vi "jrg_writeeodfile.vi"(0 "Time":string="12:00:00", 1 "Date":string="06/09/14", 2 "Path":path, 3 "Specimen":string="1", 4 "Location":string="EFish Lab", 5 "Species":string="Bennetti", 6 "UserData":sgl format="%#_13g", 7 "WaveformData":i16[](array[numeric]), 8 "NBits":i8=16, 9 "AD Range":sgl=65535.0 format="%#_13g", 10 "Version":i8, 11 "Gain":i32, 12 "NBytes":i8=2, 14 "Comments":string="Default values", 15 "Temp":string="25", 17 "Coupling":bool, 18 "Sample Rate":i32=1000, 19 "Polarity":i8) -> (13 "Path Out":path)   [LabVIEW 2014]
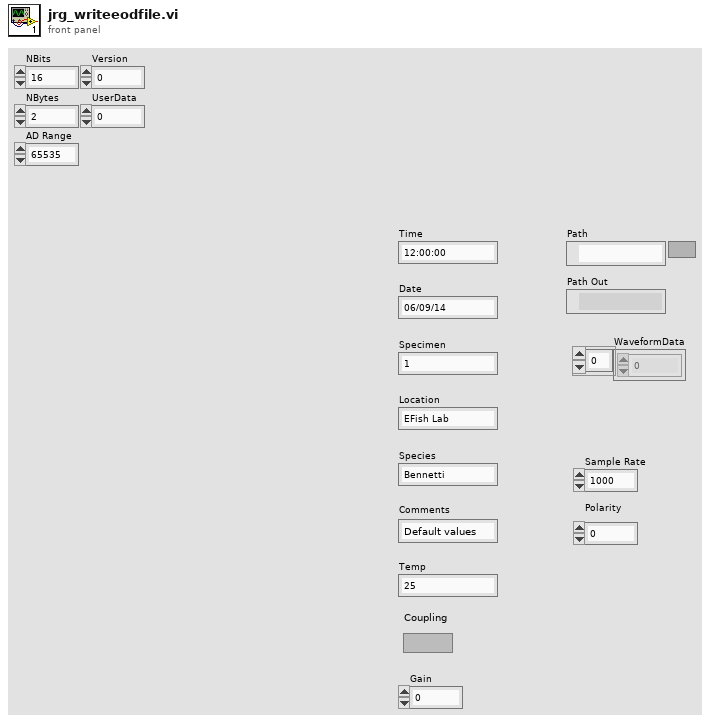
[diagram p1: front panel]
types:
  T1 = enum16{"big-endian, network order", "native, host order", "little-endian"}
  T2 = enum16{"open", "replace", "create", "open or create", "replace or create", "replace or create with confirmation"}
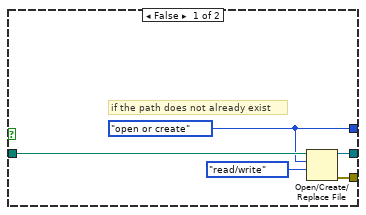
[diagram p2: hidden frame]
diagram:
  # "If File Exists,\nJump to end of file"
  # "1) If the Path is Empty:\n\na. Open file dialog\nb. Pick File Location\n\n2) If Path already exists\n\na. Open File\n\n3) If Path doesn't exist\n\na. Create File\n\n4) If Path is Full and Exists:\na. Open the file\n\n5) If Path is Full and doesn't exist\na. Create the file"
  # "Waveform Description Parameters are concatenated with prefixes:\nTime : Time of Recording\nDate: Date of Recording\nSpecimen: Specimen Number\nSpecies: Putative Species ID\nLocation: Locality Code\nComments: Further Description\nTemp: Temperature at Recording Time\nGain: Gain of Amplifier\nCoupling: AC or DC coupling\nPolarity: Inverted or Normal\n\nRecording Parameters are Gathered from Software:\nSampling Rate: Sampling Rate of A/D Converter\nNbits:\nNbytes:\nADRange:"
  n1 = Empty String/Path?(string/path="Path") -> (empty?=w22:bool)
  n2 = case shown="True" w22 {
    tunnel: "Path" -> [w34 w39]
    tunnel: [w33 w42] -> w25
    tunnel: [w32 w41] -> w27
    tunnel: [w31 w44] -> w26
    frame False {
      w31 = T2."open or create" ("operation (0:open)")
      # "if the path does not already exist"
      n3 = Open/Create/Replace File(file path (use dialog)=w34, operation (0:open)=w31, access (0:read/write)=enum16{"read/write", "read-only", "write-only"}."read/write") -> (refnum out=w33:refnum<file>, error out=w32:errorcluster)  [unwired: 3 in, 1 out]
    }
    frame True {
      # "if the path already exists"
      n4 = File Dialog(7:"Select Path", 9:"New EOD", 11:w39) -> (0:w40:errorcluster, 2:w47:bool, 3:w43:path)  [unwired: 4 in, 1 out]
      n5 = Select(t=T2."open" ("operation (0:open)"), s=w47, f=T2."create" ("operation (0:open)")) -> (s? t:f=w44:T2)
      n6 = Open/Create/Replace File(file path (use dialog)=w43, error in=w40, operation (0:open)=T2."create", access (0:read/write)=enum16{"read/write", "read-only", "write-only"}."read/write") -> (refnum out=w42:refnum<file>, error out=w41:errorcluster)  [unwired: 2 in, 1 out]
    }
  }
  n7 = call "jrg_eod_file_position.vi"("error in (no error)"=w27, "operation"=w26, "Refnum in"=w25) -> ("error out"=w11:errorcluster, "Refnum out"=w12:refnum<file>)  [unwired: 7 in]
  n8 = call "jrg_concatenate_wavetext.vi"("Specimen"="Specimen", "Date"="Date", "Time"="Time", "Temp"="Temp", "Species"="Species", "Location"="Location", "Comments"="Comments") -> ("concatenated string"=w9:string)  [unwired: 8 in]
  n9 = Array Size(array="WaveformData") -> (size(s)=w1:i32)
  n10 = call "jrg_binary_write.vi"("Byte Stream File in"=w12, "nPts"=w1, "EODText"=w9, "WaveformData"="WaveformData", "prepend array or string size? (T)"=FALSE, "error in (no error)"=w11, "AD Range"="AD Range", "NBytes"="NBytes", "UserData"="UserData", "NBits"="NBits", "Sample Rate"="Sample Rate", "byte order (0:big-endian, network order)"=T1."native, host order", "Polarity"="Polarity", "Version"="Version") -> ("Byte Stream File out"=w13:refnum<file>, "error out"=w14:errorcluster)  [unwired: 4 in]
  n11 = Close File(refnum=w13, error in=w14) -> (path=→"Path Out":path, error out=w29:errorcluster)
  n12 = call <vilib>:"Simple Error Handler.vi"("error in (no error)"=w29) -> ()  [unwired: 4 in, 5 out]
